vi "Read Controller Config.vi"(8 "error in (no error)":errorcluster, 11 "Panel Form Controller in":refnum<class "Panel Form Controller.lvclass">) -> (0 "error out":errorcluster, 2 "Controller Config":refnum<class "Panel Form Controller Configuration.lvclass">, 3 "Panel Form Controller out":refnum<class "Panel Form Controller.lvclass">)   [LabVIEW 2020, in "Panel Form Controller.lvlib" / "Panel Form Controller.lvclass"]
uses:
  Panel Form Controller.lvclass
  Controller Configuration/Panel Form Controller Configuration.lvclass
  Panel Form Controller.lvclass/Panel Form Controller.ctl
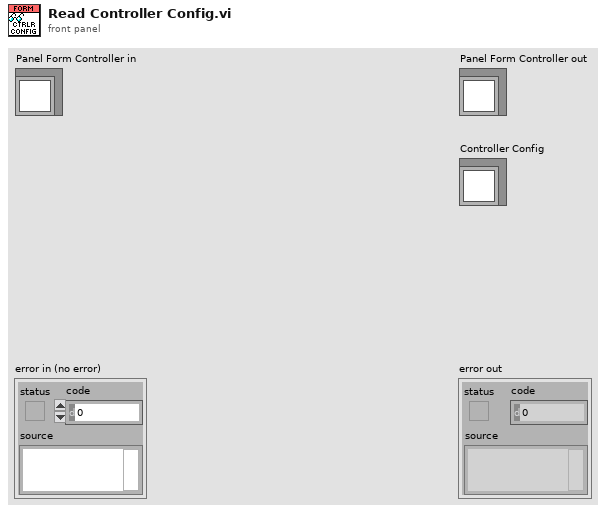
[diagram p1: front panel]
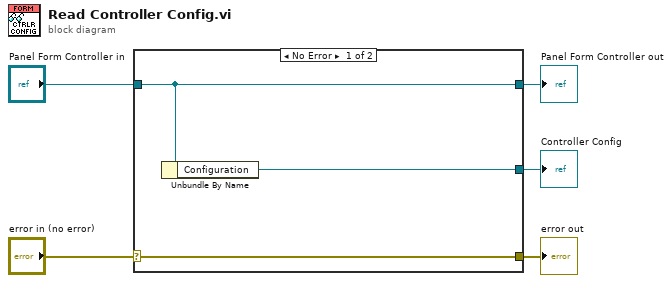
[diagram p0: block diagram]
diagram:
  n1 = case shown="No Error" "error in (no error)" {
    selector: "error in (no error)" -> [w8 w9]
    tunnel: [w8 w9] -> w4
    tunnel: [w7 w10] -> w2
    tunnel: "Panel Form Controller in" -> [w7 w10]
    tunnel: [w6 _] -> w1
    frame No Error {
      n2 = Unbundle By Name(w7) -> ("Configuration"=w6:refnum<class "Panel Form Controller Configuration.lvclass">)
    }
    frame Error {
    }
  }
  "error out" <- w4
  "Panel Form Controller out" <- w2
  "Controller Config" <- w1
